vi "current to counts.vi"(0 "Charge State":dbl=7.0, 1 "Stable Current 2":dbl, 2 "ss ratio":dbl, 3 "Stable Current 1":dbl, 4 "Live Time":dbl, 5 "ss ratio":u16(ring) items=["other", "36Cl"]) -> (7 "Stable Counts":dbl)   [LabVIEW 2016]
doc: "This vi takes the 2 stable current measureements and converts the average currents into counts"
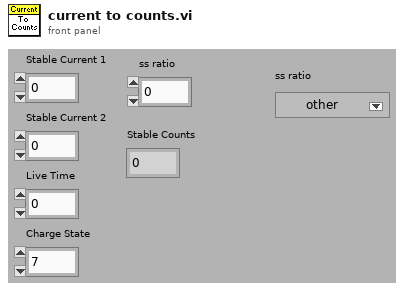
[diagram p1: front panel]
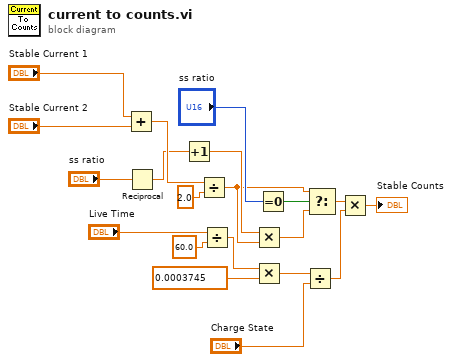
[diagram p0: block diagram]
diagram:
  n1 = Add(x="Stable Current 1", y="Stable Current 2") -> (x+y=w18:dbl)
  n2 = Reciprocal(x="ss ratio") -> (1/x=w6:dbl)
  n3 = Increment(x=w6) -> (x+1=w8:dbl)
  n4 = Divide(x=w18, y=2.0) -> (x/y=w3:dbl)
  n5 = Divide(x="Live Time", y=60.0) -> (x/y=w9:dbl)
  n6 = Multiply(x=w8, y=w3) -> (x*y=w2:dbl)
  n7 = Multiply(x=w9, y=0.0003745) -> (x*y=w12:dbl)
  n8 = Equal To 0?(x="ss ratio") -> (x = 0?=w4:bool)
  n9 = Divide(x=w12, y="Charge State") -> (x/y=w14:dbl)
  n10 = Select(t=w3, s=w4, f=w2) -> (s? t:f=w1:dbl)
  n11 = Multiply(x=w1, y=w14) -> (x*y=→"Stable Counts":dbl)
